vi "PH_ImageOperator.Set Energy.vi"(0 "i ref in":refnum<vi>, 5 "error in (no error)":errorcluster) -> (14 "i ref out":refnum<vi>, 19 "error out":errorcluster)   [LabVIEW 2014, in "PH_ImageOperator.lvlib"]
doc: "This VI calculates the energy measurement and sets it (in case of a change) to own attributes and the GUI element."
uses:
  PH_ImageOperator.lvlib
  PH_Basics/PH_Image_Common/PH_Image_Common.lvlib
  PH_Basics/PH_Common/PH_Common.lvlib
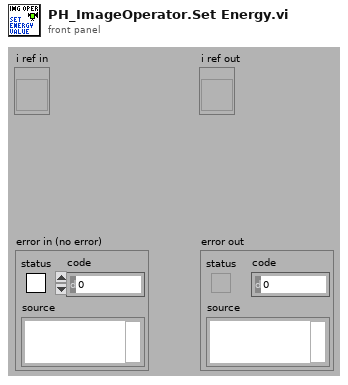
[diagram p1: front panel]
types:
  T1 = typedef "PH_ImageOperator.lvlib/PH_ImageOperator.i attribute.ctl" = cluster{"GUI Refs":cluster{"Delete":refnum<vi>, "Calibration status":refnum<vi>, "BI subtracted":refnum<vi>, "calc Energy":refnum<vi>, "Energy: expected value":refnum<vi>, "Energy: Tolerance":refnum<vi>, "Energy calculated":refnum<vi>, "Energy":refnum<vi>, "calc Beam Anal":refnum<vi>, "Maj Diam 1/esquare":refnum<vi>, "Min Diam 1/esquare":refnum<vi>, "Azi Angle":refnum<vi>, "Min/Maj Diam esquare":refnum<vi>, "Beam analysed":refnum<vi>, "CoG - x":refnum<vi>, "CoG - y":refnum<vi>, "BA: Method":refnum<vi>, "BA: Steps":refnum<vi>, "BA: Factor":refnum<vi>, "calc Traces":refnum<vi>, "Traces: Fit Gauss":refnum<vi>, "Traces calculated":refnum<vi>, "Maj FWHM":refnum<vi>, "Min FWHM":refnum<vi>, "Major Trace":refnum<vi>, "Minor Trace":refnum<vi>, "Maj Fit Order":refnum<vi>, "Min Fit Order":refnum<vi>, "Position calculated":refnum<vi>, "Position":refnum<vi>, "Type":refnum<vi>, "Center":refnum<vi>, "exp - X":refnum<vi>, "exp - Y":refnum<vi>, "Tolerance":refnum<vi>, "f":refnum<vi>, "M":refnum<vi>, "D":refnum<vi>, "q":refnum<vi>, "Dummy Method":refnum<vi>, "Dummy Type":refnum<vi>, "Global On":refnum<vi>, "Traces: No offset":refnum<vi>, "Maj 99%":refnum<vi>, "Min 99%":refnum<vi>, "GUI FF Image":refnum<vi>, "calc Fill Factor":refnum<vi>, "FF calculated":refnum<vi>, "Fill Factor: Filter?":refnum<vi>, "FF: Damage Threshold":refnum<vi>, "FF: Threshold":refnum<vi>, "FF: max allow. Energy":refnum<vi>, "FF: Fillfactor":refnum<vi>, "Calibration data":refnum<vi>}, "List of GUIs":string[], "Calibration":cluster{"Status":T2, "Calibration data":T3, "Calibration Data File":path}, "Final Image":cluster{"BI Subtraction Failure":bool}, "Energy":cluster{"on":bool, "expected value [mJ]":dbl, "Tolerance [%]":dbl, "State":T2, "Energy [mJ]":dbl, "Unit":string, "calculated @":timestamp}, "Beam Analysis":cluster{"on":bool, "Data":T4, "Method":bool, "Steps":i32, "Factor":i32, "ROI":cluster{"Left":i32, "Top":i32, "Right":i32, "Bottom":i32}, "analysed @":timestamp}, "Trace Analysis":cluster{"on":bool, "Fit on":bool, "Maj FWHM":dbl, "Min FWHM":dbl, "Maj Fit Order":i32, "Min Fit Order":i32, "No Offset":bool, "Maj 99%":dbl, "Min 99%":dbl, "Traces":cluster{"XScaleName":string, "Y Scale Minimum":sgl, "Y Scale Maximum":sgl, "X Scale Minimum":sgl, "X Scale Maximum":sgl, "Traces":cluster{"Index":sgl[], "Trace":dbl[]}[]}[], "analysed @":timestamp}, "Position Analysis":cluster{"on":bool, "exp - X":i32, "exp - Y":i32, "focal length [mm]":dbl, "Magnification":dbl, "Delta":dbl, "Theta":dbl, "Tolerance":dbl, "Type":bool, "analysed @":timestamp}, "Fill Factor":cluster{"on":bool, "Filter on?":bool, "Threshold":dbl, "Damage Threshold [J/cm²]":dbl, "Fillfactor":dbl, "Max. allowed Energy [J]":dbl, "calculated @":timestamp}, "Statistician Service ID":i32, "Images":cluster{"Background":T5, "OP":T5, "GUI":T5, "BA: ROI":T5, "Trace: Turn":T5, "FF: Main":T5, "FF: Help":T5, "PSDB: BG":T5, "PSDB: OP":T5, "PSDB: FF":T5}}
  T2 = typedef "PH_StatusHandler.lvlib/PH_StatusHandler.Status.ctl" = i16
  T3 = typedef "PH_ImageCalibrator.lvlib/PH_ImageCalibrator.Calibration Data.ctl" = cluster{"Date":string, "Time":string, "Cam Settings":cluster{"Cam ID":string, "Gain":dbl, "Brightness":dbl, "Shutter":dbl, "Cam Error":bool, "Mode":i32}, "Background Image":cluster{"Image":dbl[][], "Image Error":bool}, "Linear Calibration":cluster{"Calibration Factor":dbl, "not mm or mrad":bool}, "Energy Calibration":cluster{"Calibration Factor":dbl, "no mJ":bool}}
  T4 = typedef "PH_ImageOperator.lvlib/PH_ImageOperator.Beam Analysis Data.ctl" = cluster{"CoG-x":sgl, "CoG-y":sgl, "Maj Dim":dbl, "Min Dim":dbl, "Ellipticity":dbl, "Azimuth Angle [rad]":dbl, "Azi Angle rel to Maj?":bool}
  T5 = typedef "IMAQ Image.ctl" = refnum<image>
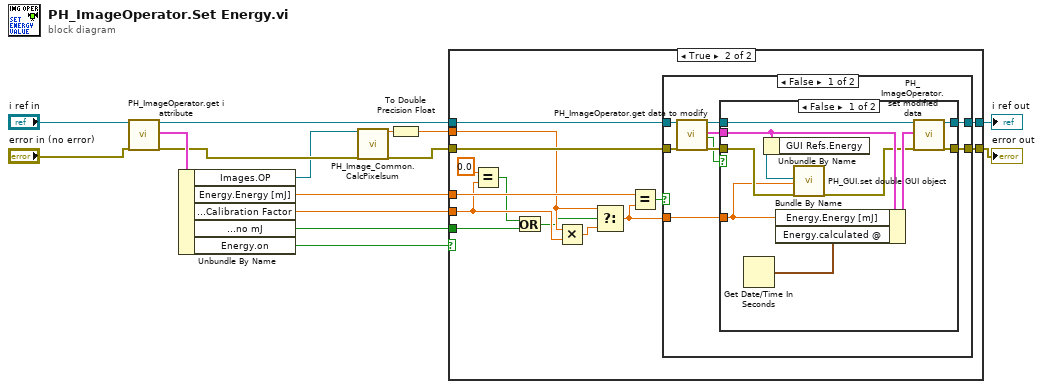
[diagram p0: block diagram]
diagram:
  n1 = call "PH_ImageOperator.get i attribute.vi"("i ref in"="i ref in", "error in (no error)"="error in (no error)") -> ("i ref out"=w11:refnum<vi>, "i attribute"=w10:T1, "error out"=w6:errorcluster)  [unwired: 15 in]
  n2 = Unbundle By Name(w10) -> ("Images.OP"=w1:T5, "Energy.Energy [mJ]"=w15:dbl, "Calibration.Calibration data.Energy Calibration.Calibration Factor"=w12:dbl, "Calibration.Calibration data.Energy Calibration.no mJ"=w2:bool, "Energy.on"=w3:bool)
  n3 = call "PH_Image_Common.CalcPixelsum.vi"("Image"=w1, "error in (no error)"=w6) -> ("Pixel Sum"=w4:sgl, "error out"=w5:errorcluster)  [unwired: 16 in]
  n4 = To Double Precision Float(number=w4) -> (double precision float=w7:dbl)
  n5 = case shown="True" w3 {
    tunnel: w11 -> [w17 w31]
    tunnel: w12 -> [_ w22]
    tunnel: w5 -> [w16 w30]
    tunnel: [w17 w29] -> w13
    tunnel: [w16 w28] -> w14
    tunnel: w15 -> [_ w27]
    tunnel: w7 -> [_ w23]
    tunnel: w2 -> [_ w19]
    frame False {
    }
    frame True {
      n6 = Equal?(x=0.0, y=w22) -> (x = y?=w20:bool)
      n7 = Or(x=w20, y=w19) -> (x .or. y?=w18:bool)
      n8 = Multiply(x=w23, y=w22) -> (x*y=w25:dbl)
      n9 = Select(t=w23, s=w18, f=w25) -> (s? t:f=w24:dbl)
      n10 = Equal?(x=w27, y=w24) -> (x = y?=w26:bool)
      n11 = case shown="False" w26 {
        tunnel: w31 -> [w37 w54]
        tunnel: w30 -> [w36 w53]
        tunnel: [w35 w54] -> w29
        tunnel: [w34 w53] -> w28
        tunnel: w24 -> [w32 _]
        frame False {
          n12 = call "PH_ImageOperator.get data to modify.vi"("i ref in"=w37, "error in (no error)"=w36) -> ("i ref out"=w39:refnum<vi>, "i attribute"=w38:T1, "timed out"=w33:bool, "error out"=w40:errorcluster)  [unwired: 14 in]
          n13 = case shown="False" w33 {
            tunnel: w40 -> [w44 w51]
            tunnel: w39 -> [w50 w52]
            tunnel: [w49 w52] -> w35
            tunnel: [w48 w51] -> w34
            tunnel: w38 -> [w47 _]
            tunnel: w32 -> [w42 _]
            frame False {
              n14 = Get Date/Time In Seconds() -> (seconds since 1Jan1904=w41:timestamp)
              n15 = Unbundle By Name(w47) -> ("GUI Refs.Energy"=w45:refnum<vi>)
              n16 = Bundle By Name(cluster=w47, "Energy.Energy [mJ]"=w42, "Energy.calculated @"=w41) -> (w46:T1)
              n17 = call "PH_GUI.set double GUI object.vi"("GUI object Ref"=w45, "value"=w42, "error in (no error)"=w44) -> ("error out"=w43:errorcluster)  [unwired: 16 in]
              n18 = call "PH_ImageOperator.set modified data.vi"("i ref in"=w50, "i attribute"=w46, "error in (no error)"=w43) -> ("i ref out"=w49:refnum<vi>, "error out"=w48:errorcluster)  [unwired: 15 in]
            }
            frame True {
            }
          }
        }
        frame True {
        }
      }
    }
  }
  "error out" <- w14
  "i ref out" <- w13
